vi "SDCP SMF Rx Logger - Notifier and Queue FGV (version 1.1).vi"(0 "Commands":T1(ring), 5 "Notification value in":bool, 11 "error in (no error)":errorcluster) -> (4 "Notifier out":refnum<notifier>, 6 "Notifier value output":bool, 10 "Queue out":refnum<queue>, 13 "Remaining elements":i32, 15 "error out":errorcluster)   [LabVIEW 2020]
uses:
  Typedefs/SDCP SMF logger - SMF with timestamp.ctl
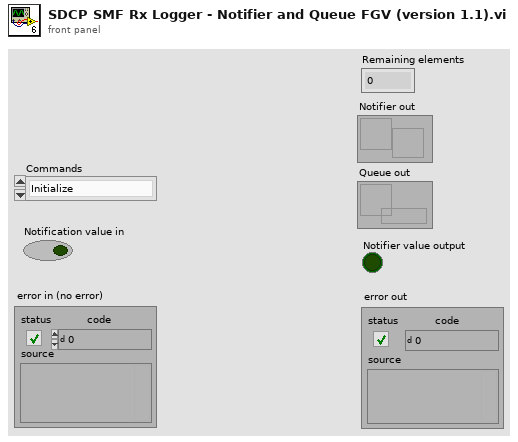
[diagram p1: front panel]
types:
  T1 = enum16{"Initialize", "Read", "Write", "Deinitialize"}
  T2 = typedef "SDCP SMF logger - SMF with timestamp.ctl" = cluster{"Bytes":u8[], "Checksum":bool, "Time (ms)":u32, "Tx/Rx":string}
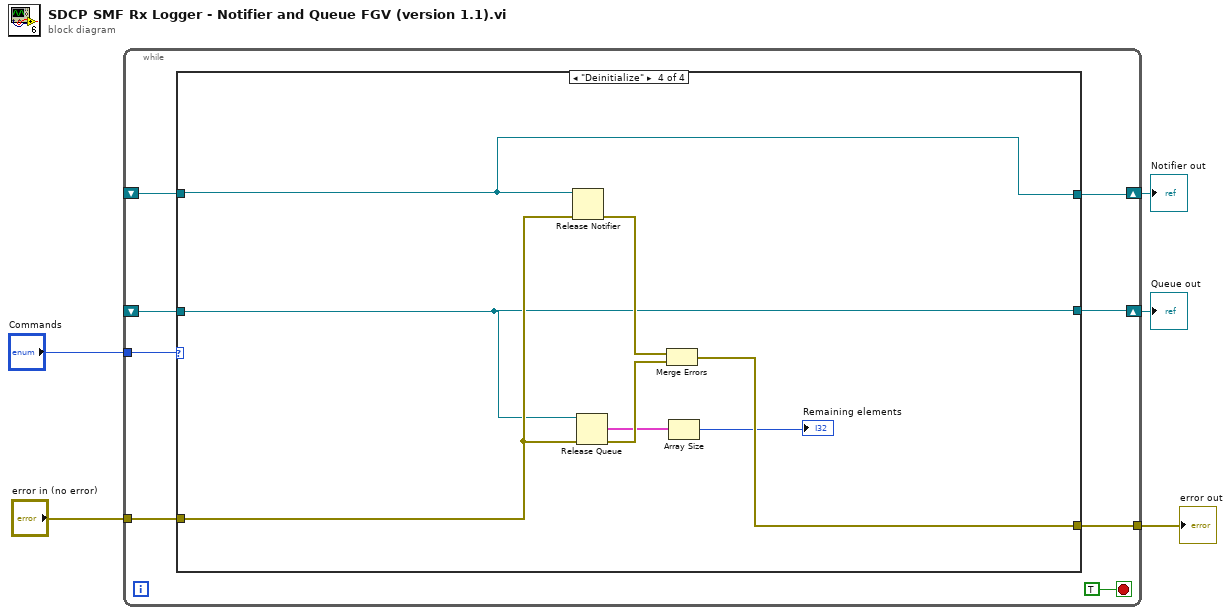
[diagram p0: block diagram]
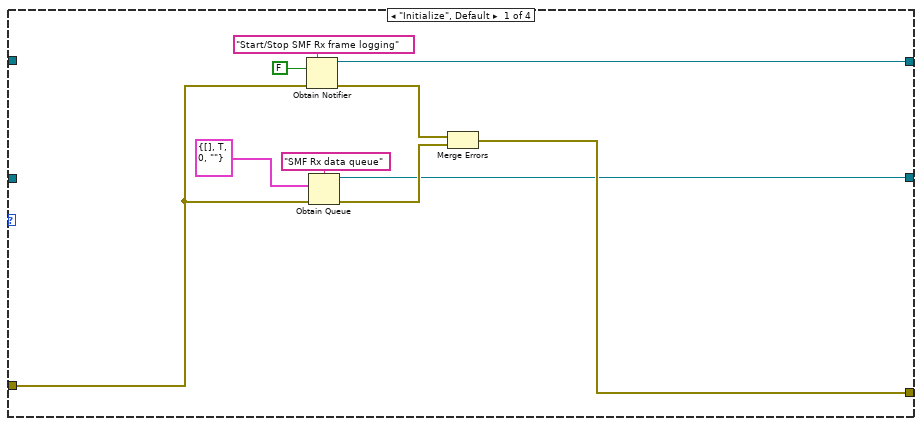
[diagram p2: hidden frame]
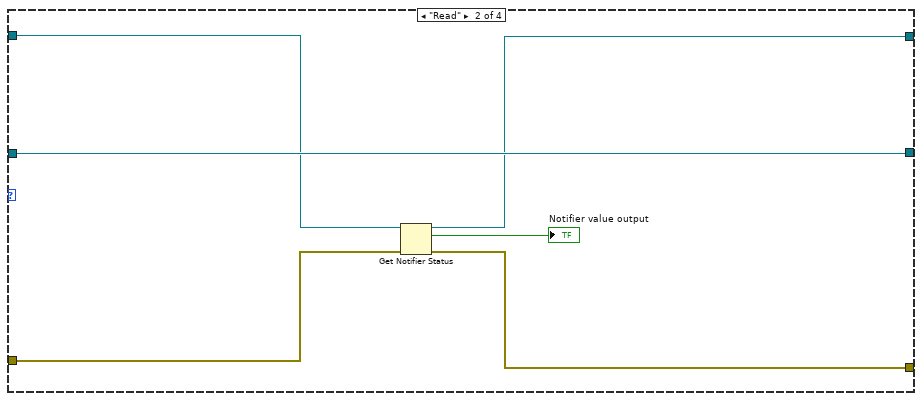
[diagram p3: hidden frame]
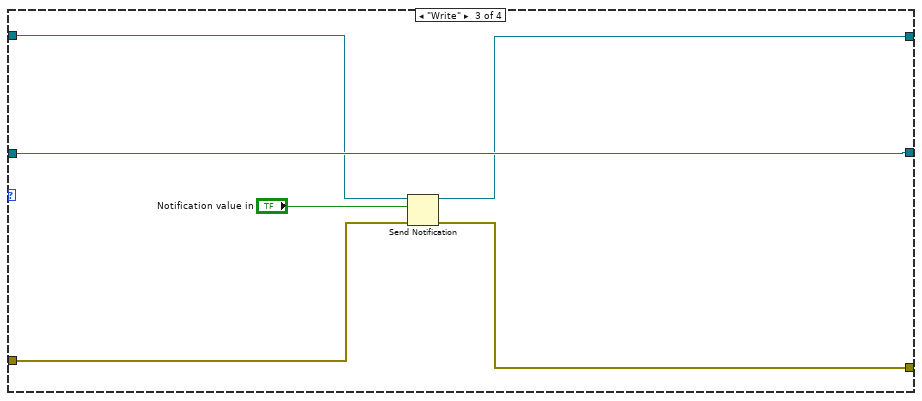
[diagram p4: hidden frame]
diagram:
  n1 = while {
    tunnel: "Commands" -> [w12]
    tunnel: "error in (no error)" -> [w11]
    shift-right: [w10] -> w3
    shift-left: _ -> [w6]
    tunnel: [w9] -> w2
    shift-right: [w8] -> w1
    shift-left: _ -> [w7]
    stop <- TRUE stop-if-true
    n2 = case shown="\"Deinitialize\"" w12 {
      tunnel: w11 -> [w20 w28 w31 w42]
      tunnel: [w21 w26 w33 w43] -> w10
      tunnel: [w15 w25 w30 w39] -> w9
      tunnel: [w14 w29 w35 w36] -> w8
      tunnel: w7 -> [_ w29 w35 w36]
      tunnel: w6 -> [_ w27 w34 w43]
      frame "Initialize", Default {
        n3 = Obtain Notifier(name (unnamed)="Start/Stop SMF Rx frame logging", notification data type=FALSE, error in (no error)=w20) -> (notifier out=w21:refnum<notifier>, error out=w17:errorcluster)  [unwired: 1 in, 1 out]
        n4 = Obtain Queue(name (unnamed)="SMF Rx data queue", element data type=T2 {"Bytes"=[], "Checksum"=TRUE, "Time (ms)"=0, "Tx/Rx"=""} ("SMF with timestamp"), error in (no error)=w20) -> (queue out=w14:refnum<queue>, error out=w16:errorcluster)  [unwired: 2 in, 1 out]
        n5 = Merge Errors(w17, w16) -> (w15:errorcluster)
      }
      frame "Read" {
        n6 = Get Notifier Status(notifier=w27, error in (no error)=w28) -> (notifier out=w26:refnum<notifier>, current notification=→"Notifier value output":bool, error out=w25:errorcluster)  [unwired: 2 out]
      }
      frame "Write" {
        n7 = Send Notification(notification="Notification value in", notifier=w34, error in (no error)=w31) -> (notifier out=w33:refnum<notifier>, error out=w30:errorcluster)
      }
      frame "Deinitialize" {
        n8 = Release Notifier(notifier=w43, error in (no error)=w42) -> (error out=w41:errorcluster)  [unwired: 1 in, 2 out]
        n9 = Release Queue(queue=w36, error in (no error)=w42) -> (remaining elements=w38:T2[], error out=w40:errorcluster)  [unwired: 1 in, 1 out]
        n10 = Merge Errors(w41, w40) -> (w39:errorcluster)
        n11 = Array Size(array=w38) -> (size(s)=→"Remaining elements":i32)
      }
    }
  }
  "error out" <- w2
  "Notifier out" <- w3
  "Queue out" <- w1
